vi "Reset AO Channels.vi"(8 "error in (no error)":errorcluster) -> (0 "error out":errorcluster)   [LabVIEW 2019, in "Reset Hardware Engine.lvlib"]
uses:
  Reset Hardware Engine.lvlib
  <vilib>/DAQmx/write.llb/DAQmx Write (Analog 1D DBL NChan 1Samp).vi
  <vilib>/DAQmx/create/channels.llb/DAQmx Create Channel (AO-Voltage-Basic).vi
  <vilib>/DAQmx/miscellaneous.llb/DAQmx Fill In Error Info.vi
  <resource>/objmgr/daqmx.rc
  <vilib>/NI VeriStand/Custom Device Tools/Custom Device Utility Library/Custom Device Utility Library.lvlib
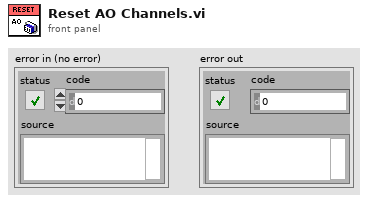
[diagram p1: front panel]
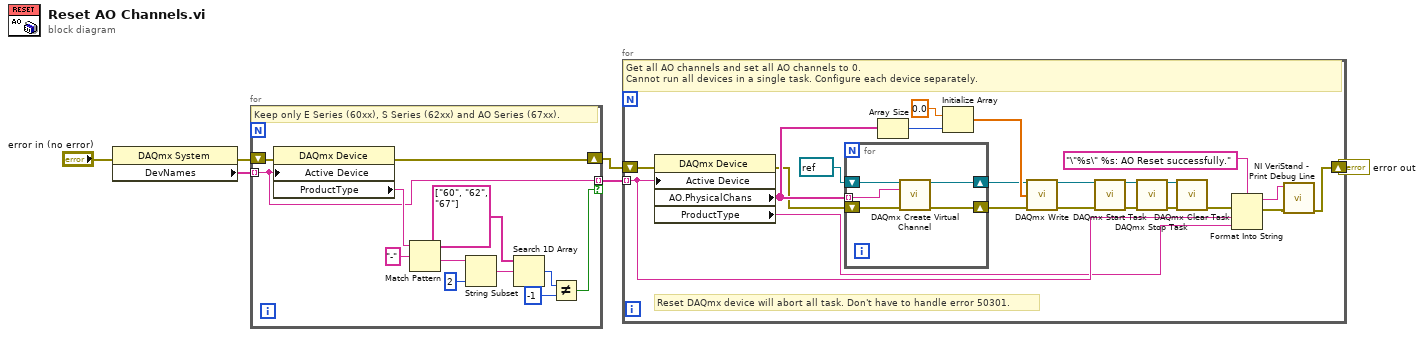
[diagram p0: block diagram]
diagram:
  n1 = property on="Property Node" class="DAQmx System"(error in="error in (no error)") -> (error out=w2:errorcluster, "DevNames"=w1:tag[])  [unwired: 1 in, 1 out]
  n2 = for {
    tunnel: w1 -> [w9] mode=indexing
    tunnel: [w9] -> w3 mode=indexing if=w8
    shift-right: [w7] -> w4
    shift-left: w2 -> [w18]
    # "Keep only E Series (60xx), S Series (62xx) and AO Series (67xx)."
    n3 = property on="Property Node" class="DAQmx Device"(error in=w18, "Active Device"=w9) -> (error out=w7:errorcluster, "ProductType"=w17:string)  [unwired: 1 in, 1 out]
    n4 = Match Pattern(string=w17, regular expression="-") -> (after substring=w15:string)  [unwired: 1 in, 3 out]
    n5 = String Subset(string=w15, length (rest)=2 ("length (rest)")) -> (substring=w12:string)  [unwired: 1 in]
    n6 = Search 1D Array(1D array=string[] ["60", "62", "67"], element=w12) -> (index of element=w11:i32)  [unwired: 1 in]
    n7 = Not Equal?(x=w11, y=-1) -> (x != y?=w8:bool)
  }
  n8 = for {
    tunnel: w3 -> [w23] mode=indexing
    shift-right: [w19] -> w6
    shift-left: w4 -> [w40]
    # "Reset DAQmx device will abort all task. Don't have to handle error 50301."
    # "Get all AO channels and set all AO channels to 0.\nCannot run all devices in a single task. Configure each device separately."
    n9 = property on="Property Node" class="DAQmx Device"(error in=w40, "Active Device"=w23) -> (error out=w28:errorcluster, "AO.PhysicalChans"=w29:tag[], "ProductType"=w22:string)  [unwired: 1 in, 1 out]
    n10 = for {
      shift-right: [w45] -> w32
      shift-left: refnum<k21> refnum ("task out") -> [w43]
      tunnel: w29 -> [w42] mode=indexing
      shift-right: [w44] -> w33
      shift-left: w28 -> [w41]
      n11 = call-poly <vilib>:"DAQmx Create Virtual Channel.vi"("task in"=w43, "physical channels"=w42, "error in"=w41) -> ("task out"=w45:refnum<k21>, "error out"=w44:errorcluster)  [unwired: 11 in]
    }
    n12 = Array Size(array=w29) -> (size(s)=w38:i32)
    n13 = Initialize Array(0.0 ("element"), w38) -> (w39:dbl[])
    n14 = call-poly <vilib>:"DAQmx Write.vi"("task/channels in"=w32, "data"=w39, "error in"=w33) -> ("task out"=w35:refnum<k21>, "error out"=w36:errorcluster)  [unwired: 10 in, 1 out]
    n15 = call <vilib>:"DAQmx Start Task.vi"("task/channels in"=w35, "error in"=w36) -> ("task out"=w26:refnum<k21>, "error out"=w37:errorcluster)  [unwired: 12 in]
    n16 = call <vilib>:"DAQmx Stop Task.vi"("task/channels in"=w26, "error in"=w37) -> ("task out"=w27:refnum<k21>, "error out"=w34:errorcluster)  [unwired: 12 in]
    n17 = call <vilib>:"DAQmx Clear Task.vi"("task in"=w27, "error in"=w34) -> ("error out"=w24:errorcluster)  [unwired: 13 in]
    n18 = Format Into String(format string="\"%s\" %s: AO Reset successfully.", error in=w24, w23, w22) -> (resulting string=w20:string, error out=w21:errorcluster)  [unwired: 1 in]
    n19 = call <vilib>:"NI VeriStand - Print Debug Line.vi"("error in (no error)"=w21, "Message"=w20) -> ("error out"=w19:errorcluster)  [unwired: 9 in]
  }
  "error out" <- w6
